vi "Read Root Lifetime.vi"(11 "TEMPLATE Actor in":refnum<class "TEMPLATE Actor.lvclass">) -> (2 "Root Lifetime":refnum<data-value>)   [LabVIEW 2020, in "_Template.lvlib" / "Templates.lvlib" / "TEMPLATE jettl Actor.lvlib" / "TEMPLATE Actor.lvlib" / "TEMPLATE Actor.lvclass"]
uses:
  TEMPLATE Actor.lvclass
  TEMPLATE Actor.lvclass/TEMPLATE Actor.ctl
  jettl/jettl/jettl.lvlib
  jettl/jettl/Actor/Actor.lvclass
  jettl/jettl/Root Lifetime.ctl
panel:
  # "This front panel should not be manipulated."
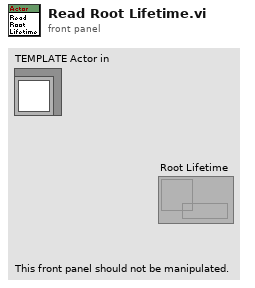
[diagram p1: front panel]
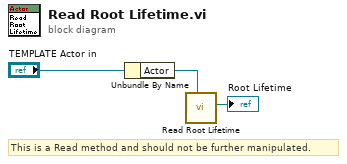
[diagram p0: block diagram]
diagram:
  # "This is a Read method and should not be further manipulated."
  n1 = Unbundle By Name("TEMPLATE Actor in") -> ("Actor"=w1:refnum<data-value>)
  n2 = call "Read Root Lifetime.vi"("Actor in"=w1) -> ("Root Lifetime"=→"Root Lifetime":refnum<data-value>)  [unwired: 10 in]
